vi "SR SIM921 Add Curve Point.vi"(5 "Sensor":dbl, 7 "Temperature":dbl, 8 "Error In":errorcluster, 9 "Curve #":u32=1, 10 "Slot":T1(ring), 11 "VISA resource name":refnum<visa-resource-name>) -> (0 "Error Out":errorcluster, 3 "VISA resource name":refnum<visa-resource-name>)   [LabVIEW 2019]
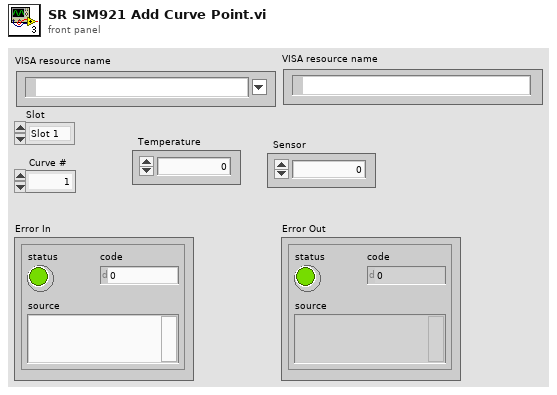
[diagram p1: front panel]
types:
  T1 = enum32{"Slot 1", "Slot 2", "Slot 3", "Slot 4", "Slot 5", "Slot 6", "Slot 7", "Slot 8"}
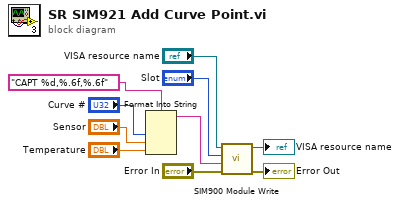
[diagram p0: block diagram]
diagram:
  n1 = Format Into String(format string="CAPT %d,%.6f,%.6f", "Curve #", "Sensor", "Temperature") -> (resulting string=w5:string)  [unwired: 2 in, 1 out]
  n2 = call "SIM900 Module Write.vi"("Error In"="Error In", "Query"=w5, "Slot"="Slot", "VISA Resource Name"="VISA resource name") -> ("Error Out"=→"Error Out":errorcluster, "dup VISA Session"=→"VISA resource name":refnum<visa-resource-name>)  [unwired: 6 in]
